vi "validate configuration.vi"(8 "error in":errorcluster, 11 "UI Reference configuration in":refnum<class "UI Reference configuration.lvclass">) -> (0 "error out":errorcluster, 3 "UI Reference configuration out":refnum<class "UI Reference configuration.lvclass">)   [LabVIEW 2013, in "UI Reference configuration.lvclass"]
doc: "This function performs validation of the configuration. This function should be safe to call at any point and should not rely on anything in the runtime environment."
uses:
  UI Reference configuration.lvclass
  <vilib>/NI/Tag Bus Module Framework/module configuration/TBM module configuration.lvclass
  UI Reference configuration.lvclass/UI Reference configuration.ctl
  Read VI name.vi
  Read VI path.vi
  <vilib>/NI/Tag Bus Module Framework/root configuration/TBM configuration.lvclass
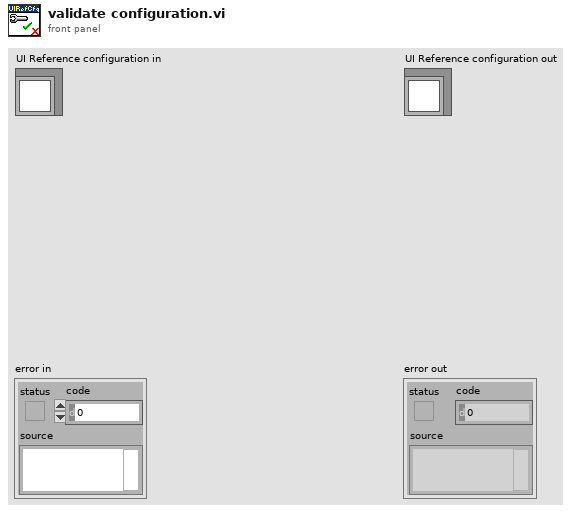
[diagram p1: front panel]
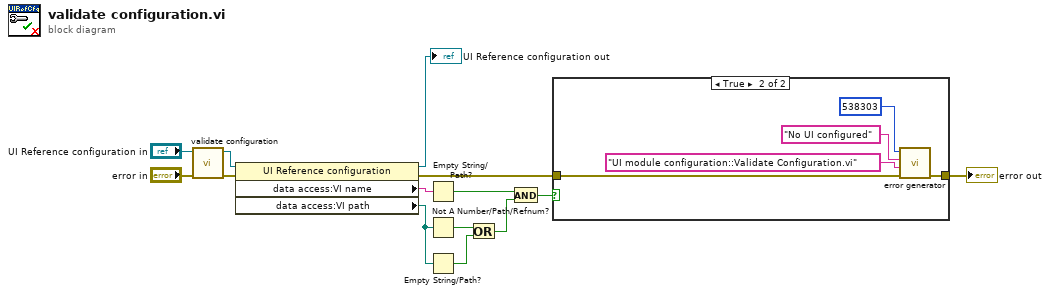
[diagram p0: block diagram]
diagram:
  n1 = call-parent "validate configuration.vi"("error in"="error in", "configuration in"="UI Reference configuration in") -> ("error out"=w14:errorcluster, "configuration out"=w11:refnum<class "UI Reference configuration.lvclass">)  [unwired: 8 in]
  n2 = property class="UI Reference configuration"(reference=w11, error in=w14) -> (reference out=→"UI Reference configuration out":refnum<class "UI Reference configuration.lvclass">, error out=w9:errorcluster, "data access:VI name"=w7:string, "data access:VI path"=w1:path)
  n3 = Empty String/Path?(string/path=w7) -> (empty?=w6:bool)
  n4 = Not A Number/Path/Refnum?(number/path/refnum=w1) -> (NaN/Path/Refnum?=w3:bool)
  n5 = Empty String/Path?(string/path=w1) -> (empty?=w4:bool)
  n6 = Or(x=w3, y=w4) -> (x .or. y?=w2:bool)
  n7 = And(x=w6, y=w2) -> (x .and. y?=w5:bool)
  n8 = case shown="True" w5 {
    tunnel: w9 -> [w15 w17]
    tunnel: [w15 w16] -> w8
    frame False {
    }
    frame True {
      n9 = call <vilib>:"error generator.vi"("error in"=w17, "source"="UI module configuration::Validate Configuration.vi", "append error message"="No UI configured", "error code (0)"=538303) -> ("error out"=w16:errorcluster)  [unwired: 7 in]
    }
  }
  "error out" <- w8
